vi "LabView360-6.vi"() -> ()   [LabVIEW 2017]
panel:
  in  "停止":bool
  out "波形图表 2":dbl(graph)
  out "波形图表":dbl(graph)
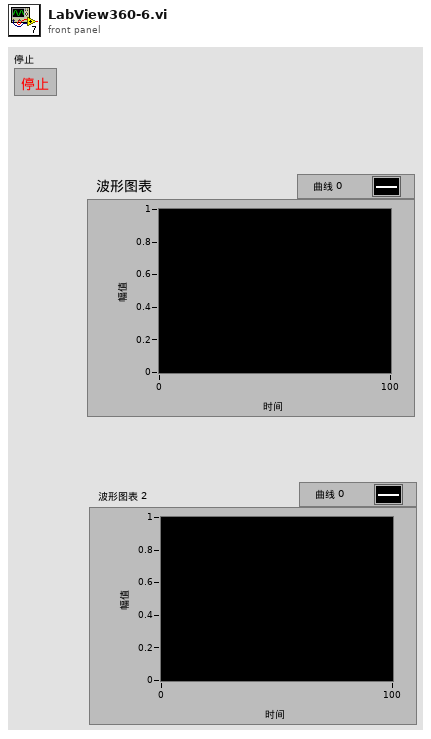
[diagram p1: front panel]
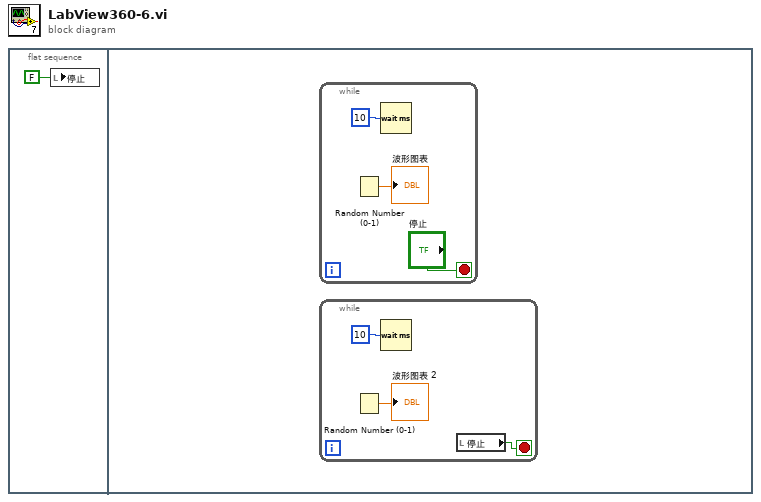
[diagram p0: block diagram]
diagram:
  n1 = flat-sequence {
    frame #0 {
      n2 = local write "停止"(FALSE ("停止")) -> ()
    }
    frame #1 {
      n3 = while {
        stop <- "停止" stop-if-true
        n4 = Random Number (0-1)() -> (number: 0 to 1=→"波形图表":dbl)
        n5 = Wait (ms)(milliseconds to wait=u32 10 ("等待时间（毫秒）")) -> ()  [unwired: 1 out]
      }
      n6 = while {
        stop <- w2 stop-if-true
        n7 = Random Number (0-1)() -> (number: 0 to 1=→"波形图表 2":dbl)
        n8 = Wait (ms)(milliseconds to wait=u32 10 ("等待时间（毫秒）")) -> ()  [unwired: 1 out]
        n9 = local read "停止"() -> (w2:bool)
      }
    }
  }
